vi "Wait (ms) With Conditional Error Input.vi"(7 "wait if error (F)":bool, 8 "error in (no error)":errorcluster, 10 "milliseconds to wait":u32=5000) -> (0 "error out":errorcluster, 2 "millisecond timer value":u32)   [LabVIEW 2020, in "varilib.lvlib"]
doc: "Waits the specified number of milliseconds and returns the value of the millisecond timer. Wiring a value of 0 to the milliseconds to wait input forces the current thread to yield control of the CPU. Vi is not executed if error in. If set, vi waits even if error is on error in input"
uses:
  varilib.lvlib
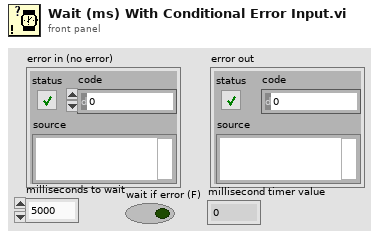
[diagram p1: front panel]
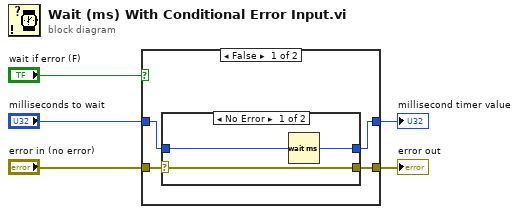
[diagram p0: block diagram]
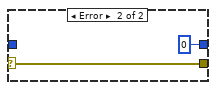
[diagram p2: hidden frame]
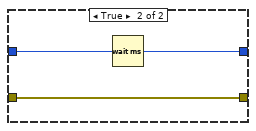
[diagram p3: hidden frame]
diagram:
  n1 = case shown="False" "wait if error (F)" {
    tunnel: "error in (no error)" -> [w9 w17]
    tunnel: [w8 w17] -> w4
    tunnel: [w7 w15] -> w3
    tunnel: "milliseconds to wait" -> [w6 w16]
    frame False {
      n2 = case shown="No Error" w9 {
        selector: w9 -> [w12 w14]
        tunnel: [w12 w14] -> w8
        tunnel: [w11 u32 0 ("millisecond timer value")] -> w7
        tunnel: w6 -> [w10 _]
        frame No Error {
          n3 = Wait (ms)(milliseconds to wait=w10) -> (millisecond timer value=w11:u32)
        }
        frame Error {
        }
      }
    }
    frame True {
      n4 = Wait (ms)(milliseconds to wait=w16) -> (millisecond timer value=w15:u32)
    }
  }
  "error out" <- w4
  "millisecond timer value" <- w3
